vi "GetLanguageFile.vi"(9 "Action":enum16{"Get", "Set"}(ring), 11 "Filename":path) -> (2 "LanguageFileContents":string, 3 "Success?":bool)   [LabVIEW 2013]
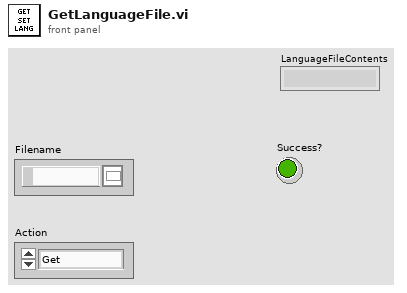
[diagram p1: front panel]
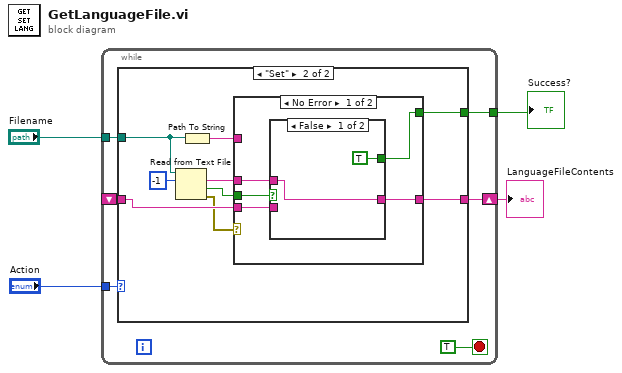
[diagram p0: block diagram]
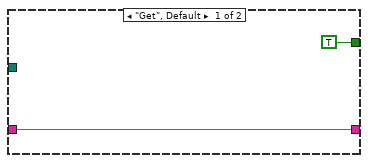
[diagram p2: hidden frame]
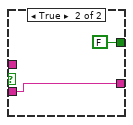
[diagram p3: hidden frame]
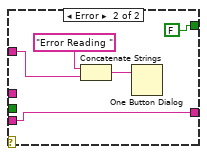
[diagram p4: hidden frame]
diagram:
  n1 = while {
    tunnel: "Action" -> [w9]
    tunnel: "Filename" -> [w8]
    shift-right: [w7] -> w1
    shift-left: _ -> [w5]
    tunnel: [w6] -> w2
    stop <- TRUE stop-if-true
    n2 = case shown="\"Set\"" w9 {
      tunnel: w8 -> [_ w15]
      tunnel: [w11 w17] -> w7
      tunnel: [TRUE w13] -> w6
      tunnel: w5 -> [w11 w19]
      frame "Get", Default {
      }
      frame "Set" {
        n3 = Read from Text File(file (use dialog)=w15, count=-1) -> (text=w18:string, cancelled=w20:bool, error out=w16:errorcluster)  [unwired: 2 in, 1 out]
        n4 = Path To String(path=w15) -> (string=w14:string)
        n5 = case shown="No Error" w16 {
          tunnel: w20 -> [w26 _]
          tunnel: w19 -> [w25 w35]
          tunnel: w18 -> [w24 _]
          tunnel: [w23 w35] -> w17
          tunnel: w14 -> [_ w32]
          tunnel: [w22 FALSE] -> w13
          frame No Error {
            n6 = case shown="False" w26 {
              tunnel: w25 -> [_ w30]
              tunnel: w24 -> [w28 _]
              tunnel: [w28 w30] -> w23
              tunnel: [TRUE FALSE] -> w22
              frame False {
              }
              frame True {
              }
            }
          }
          frame Error {
            n7 = Concatenate Strings("Error Reading ", w32) -> (w34:string)
            n8 = One Button Dialog(message=w34) -> ()  [unwired: 1 in, 1 out]
          }
        }
      }
    }
  }
  "Success?" <- w2
  "LanguageFileContents" <- w1
